vi "DecodeVireoToBotSpeak.vi"(3 "Via file":string="// Autogenerated Vireo assembly file\n// Generated on Wed Dec 18 16:11:37 2013\n\ndefine (c0, v(.UInt16 1) )\ndefine (c1, v(.UInt16 0) )\ndefine (c2, v(.UInt8 13) )\ndefine (c3, v(.Single 1000) )\n//---------------------------------------------------\n//VI Definition: Demo1.vi\ndefine (videf1, v(.VirtualInstrument, (\n    c(\n        e(.Utf8String local1)   // Reply\n        e(c(\n            e(.UInt8 n0)   // Numeric\n        ) local2)   // Info Out\n        e(.Utf8String local3)   // Reply\n        e(c(\n            e(.UInt8 n0)   // Numeric\n        ) local4)   // Info Out\n        e(.Utf8String local5)   // Reply\n    )\n    1,\n    clump(1,\n        videf2(c1 local1  c2 local2)\n        videf3( local3 local2  local4)\n        videf2(c0 local5 local4 c2 local2)\n//--- end of vi\n    )\n)))\n//---------------------------------------------------\n//VI Definition: DigitalWrite.vi\ndefine (videf2, v(.VirtualInstrument, (\n    c(\n        i(v(.UInt16 0) local4)   // State\n        o(v(.Utf8String '') local3)   // Reply\n        i(v(c(\n            e(.UInt8 n0)   // Numeric\n        ) (0 )) local1)   // Info In\n        i(v(.UInt8 0) local5)   // Port\n        o(v(c(\n            e(.UInt8 n0)   // Numeric\n        ) (0 )) local2)   // Info Out\n    )\n    c(\n        e(v(.Int32 -1) local6)\n    )\n    1,\n    clump(1,\n        Copy(local1 local2 )                      // FP Term\n//--- end of vi\n    )\n)))\n//---------------------------------------------------\n//VI Definition: VS_Wait.vi\ndefine (videf3, v(.VirtualInstrument, (\n    c(\n        i(v(.Single 1) local4)   // delay (s)\n        o(v(.Utf8String '') local3)   // Reply\n        i(v(c(\n            e(.UInt8 n0)   // Numeric\n        ) (0 )) local1)   // Info In\n        i(v(.UInt8 0) local8)   // Timer\n        o(v(c(\n            e(.UInt8 n0)   // Numeric\n        ) (0 )) local2)   // Info Out\n    )\n    c(\n        e(.Single local5)\n        e(.UInt32 local6)   // milliseconds to wait\n        e(.UInt32 local7)   // millisecond timer value\n        e(v(.Int32 -1) local9)\n    )\n    1,\n    clump(1,\n        Copy(local1 local2 )                      // FP Term\n        Mul(local4 c3 local5)\n        Convert(local5 local6)\n        WaitMilliseconds(local6)\n//--- end of vi\n    )\n)))\nenqueue (videf1)\n") -> (1 "BotSpeak":string)   [LabVIEW 2012]
panel:
  out "Array 3":string[](array[string])
  out "Params":cluster{"Constant":string, "value":string}[](array[cluster])
  out "Array":T1(array[cluster])
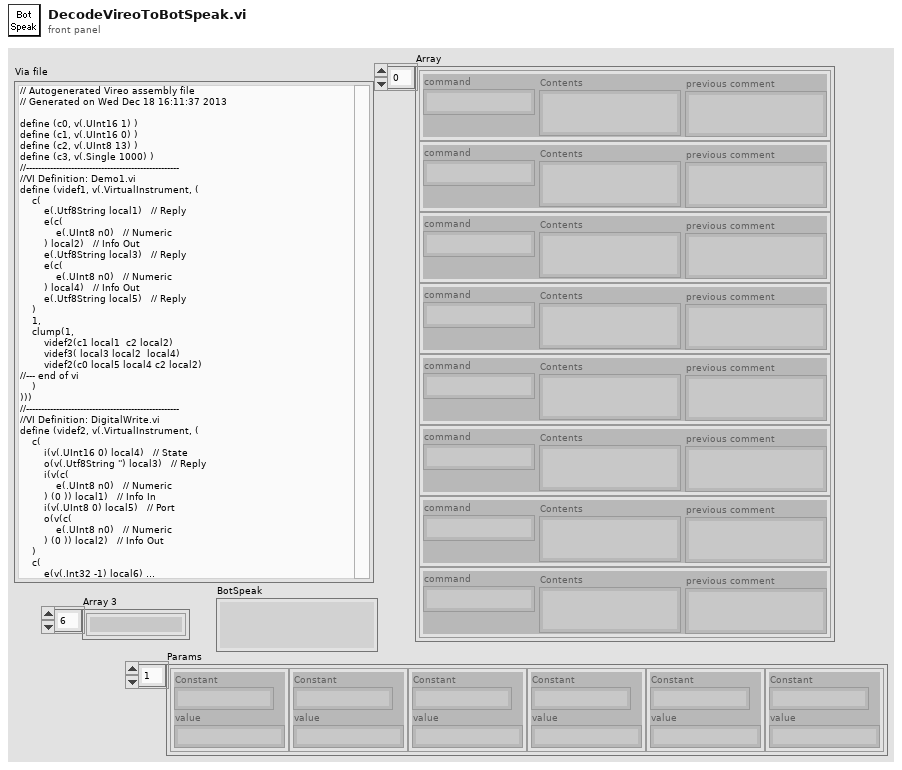
[diagram p1: front panel]
types:
  T1 = cluster{"command":string, "Contents":string, "previous comment":string}[]
  T2 = cluster{"Contents":string, "Contents 2":string}[]
  T3 = cluster{"command":string, "Contents":string, "Via file":string}
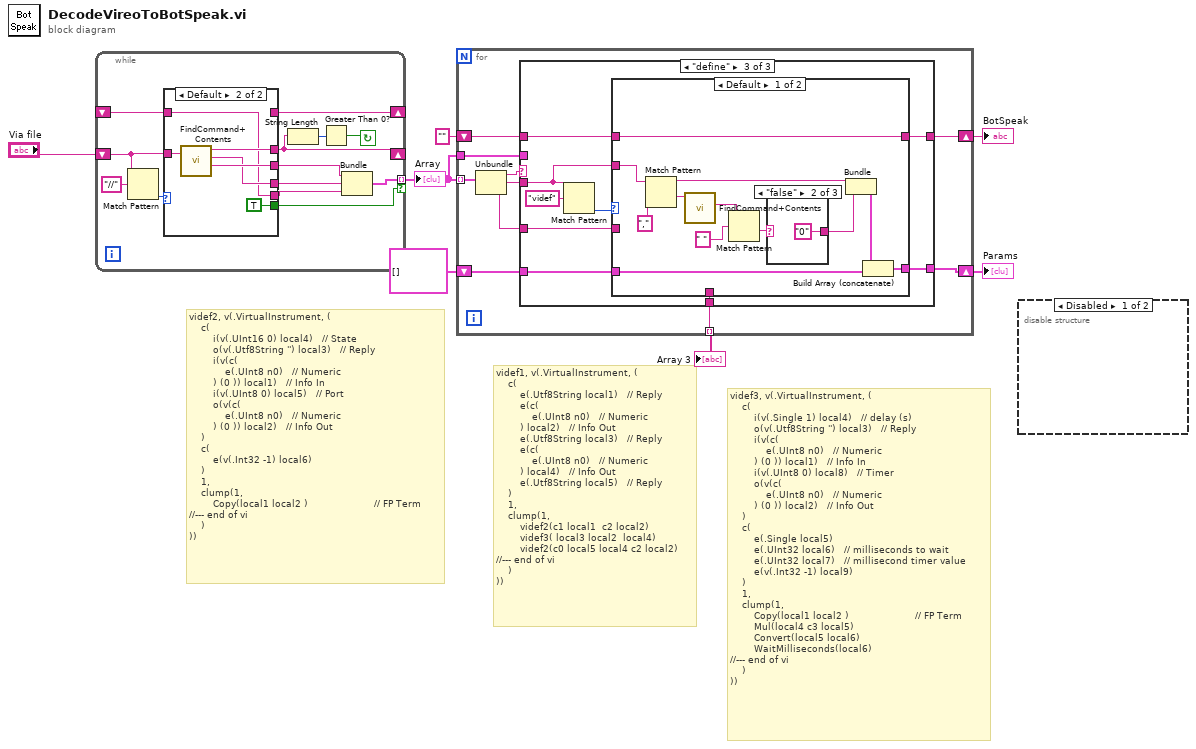
[diagram p0: block diagram]
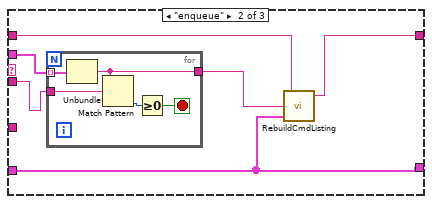
[diagram p4: hidden frame]
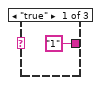
[diagram p5: hidden frame]
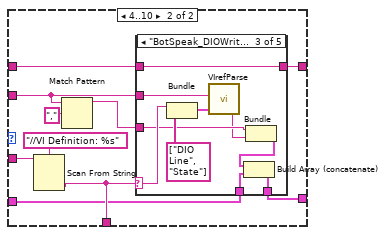
[diagram p7: hidden frame]
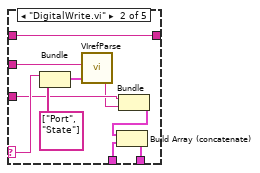
[diagram p9: hidden frame]
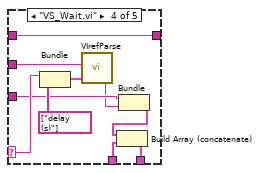
[diagram p10: hidden frame]
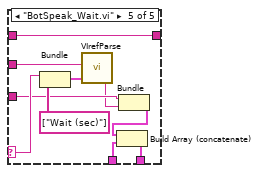
[diagram p11: hidden frame]
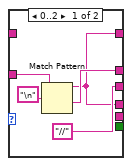
[diagram p12: hidden frame]
diagram:
  # "videf3, v(.VirtualInstrument, (\n    c(\n        i(v(.Single 1) local4)   // delay (s)\n        o(v(.Utf8String '') local3)   // Reply\n        i(v(c(\n            e(.UInt8 n0)   // Numeric\n        ) (0 )) local1)   // Info In\n        i(v(.UInt8 0) local8)   // Timer\n        o(v(c(\n            e(.UInt8 n0)   // Numeric\n        ) (0 )) local2)   // Info Out\n    )\n    c(\n        e(.Single local5)\n        e(.UInt32 local6)   // milliseconds to wait\n        e(.UInt32 local7)   // millisecond timer value\n        e(v(.Int32 -1) local9)\n    )\n    1,\n    clump(1,\n        Copy(local1 local2 )                      // FP Term\n        Mul(local4 c3 local5)\n        Convert(local5 local6)\n        WaitMilliseconds(local6)\n//--- end of vi\n    )\n))"
  # "videf1, v(.VirtualInstrument, (\n    c(\n        e(.Utf8String local1)   // Reply\n        e(c(\n            e(.UInt8 n0)   // Numeric\n        ) local2)   // Info Out\n        e(.Utf8String local3)   // Reply\n        e(c(\n            e(.UInt8 n0)   // Numeric\n        ) local4)   // Info Out\n        e(.Utf8String local5)   // Reply\n    )\n    1,\n    clump(1,\n        videf2(c1 local1  c2 local2)\n        videf3( local3 local2  local4)\n        videf2(c0 local5 local4 c2 local2)\n//--- end of vi\n    )\n))"
  # "videf2, v(.VirtualInstrument, (\n    c(\n        i(v(.UInt16 0) local4)   // State\n        o(v(.Utf8String '') local3)   // Reply\n        i(v(c(\n            e(.UInt8 n0)   // Numeric\n        ) (0 )) local1)   // Info In\n        i(v(.UInt8 0) local5)   // Port\n        o(v(c(\n            e(.UInt8 n0)   // Numeric\n        ) (0 )) local2)   // Info Out\n    )\n    c(\n        e(v(.Int32 -1) local6)\n    )\n    1,\n    clump(1,\n        Copy(local1 local2 )                      // FP Term\n//--- end of vi\n    )\n))"
  n1 = while {
    shift-right: [w20] -> _
    shift-left: "Via file" -> [w14]
    tunnel: [w15] -> w1 mode=indexing if=w9
    shift-right: [w11] -> _
    shift-left: _ -> [w10]
    stop <- w18 continue-if-true
    n2 = Match Pattern(string=w14, regular expression="//") -> (offset past match=w12:i32)  [unwired: 1 in, 3 out]
    n3 = case shown="Default" w12 {
      tunnel: [w23 w31] -> w20
      tunnel: ["//" ("regular expression") w30] -> w17
      tunnel: [w21 w29] -> w16
      tunnel: w14 -> [w25 w28]
      tunnel: [w21 _] -> w11
      tunnel: [_ w27] -> w8
      tunnel: w10 -> [_ w27]
      tunnel: [_ TRUE] -> w9
      frame 0..2 {
        n4 = Match Pattern(string=w25, regular expression="\n") -> (before substring=w21:string, after substring=w23:string)  [unwired: 1 in, 2 out]
      }
      frame Default {
        n5 = call "FindCommand+Contents.vi"("Via file in"=w28) -> ("left"=w31:string, "Contents"=w29:string, "command"=w30:string)  [unwired: 1 in, 1 out]
      }
    }
    n6 = String Length(string=w20) -> (length=w19:i32)
    n7 = Greater Than 0?(x=w19) -> (x > 0?=w18:bool)
    n8 = Bundle("command"=w17, "Contents"=w16, "Via file"=w8) -> (w15:T3)  [unwired: 1 in]
  }
  "Array" <- w1
  n9 = for {
    tunnel: w1 -> [w41] mode=indexing
    shift-right: [w36] -> w5
    shift-left: "" -> [w37]
    shift-right: [w35] -> w3
    shift-left: T2 [] -> [w34]
    tunnel: [w33] -> w2 mode=indexing
    tunnel: w1 -> [w32]
    n10 = Unbundle(w41) -> ("command"=w40:string, "Contents"=w39:string, "Via file"=w38:string)
    n11 = case shown="\"define\"" w40 {
      tunnel: w39 -> [_ w46 w58]
      tunnel: w38 -> [_ _ w61]
      tunnel: w37 -> [w43 w48 w60]
      tunnel: [w43 w49 w59] -> w36
      tunnel: [w42 w44 w57] -> w35
      tunnel: w34 -> [w42 w44 w56]
      tunnel: [_ _ w55] -> w33
      tunnel: w32 -> [_ w47 _]
      frame Default {
      }
      frame "enqueue" {
        n12 = for {
          tunnel: w47 -> [w54] mode=indexing
          tunnel: w46 -> [w53]
          tunnel: [w50] -> w45
          stop <- w51 stop-if-true
          n13 = Unbundle(w54) -> ("Contents"=w50:string)  [unwired: 2 out]
          n14 = Match Pattern(string=w50, regular expression=w53) -> (offset past match=w52:i32)  [unwired: 1 in, 3 out]
          n15 = Greater Or Equal To 0?(x=w52) -> (x >= 0?=w51:bool)
        }
        n16 = call "RebuildCmdListing.vi"("Params"=w44, "Contents"=w45, "String in"=w48) -> ("String out"=w49:string)  [unwired: 1 in, 1 out]
      }
      frame "define" {
        n17 = Match Pattern(string=w58, regular expression="videf") -> (offset past match=w62:i32)  [unwired: 1 in, 3 out]
        n18 = case shown="Default" w62 {
          tunnel: w61 -> [_ w88]
          tunnel: w60 -> [w75 w86]
          tunnel: [w75 w85] -> w59
          tunnel: w58 -> [w73 w83]
          tunnel: [w67 w79] -> w57
          tunnel: w56 -> [w66 w80]
          tunnel: [_ w84] -> w55
          frame Default {
            n19 = Match Pattern(string=w73, regular expression=",") -> (before substring=w71:string, after substring=w72:string)  [unwired: 1 in, 2 out]
            n20 = call "FindCommand+Contents.vi"("Via file in"=w72) -> ("Contents"=w70:string)  [unwired: 1 in, 3 out]
            n21 = Match Pattern(string=w70, regular expression=" ") -> (after substring=w65:string)  [unwired: 1 in, 3 out]
            n22 = case shown="\"false\"" w65 {
              selector: w65 -> [_ _ w78]
              tunnel: ["1" "0" w78] -> w64
              frame "true" {
              }
              frame "false" {
              }
              frame Default {
              }
            }
            n23 = Bundle("Contents"=w71, w64) -> (w68:cluster{"Contents":string, string})  [unwired: 1 in]
            n24 = Build Array (concatenate)(w68, w66) -> (w67:T2)
          }
          frame 4..10 {
            n25 = Scan From String(format string="//VI Definition: %s" ("regular expression"), input string=w88) -> (output 1=w84:string)  [unwired: 3 in, 3 out]
            n26 = Match Pattern(string=w83, regular expression=",") -> (before substring=w81:string)  [unwired: 1 in, 3 out]
            n27 = case shown="\"BotSpeak_DIOWrite.vi\"" w84 {
              selector: w84 -> [_ w99 w109 w119 w129]
              tunnel: w86 -> [w90 w96 w106 w116 w126]
              tunnel: [w90 w96 w106 w116 w126] -> w85
              tunnel: w83 -> [_ w100 w110 w120 w130]
              tunnel: w81 -> [_ w95 w105 w115 w125]
              tunnel: w80 -> [w89 w92 w102 w112 w122]
              tunnel: [w89 w91 w101 w111 w121] -> w79
              frame Default {
              }
              frame "DigitalWrite.vi" {
                n28 = Bundle(w99, string[] ["Port", "State"]) -> (w97:cluster{string, string[]})  [unwired: 1 in]
                n29 = call "VIrefParse.vi"("Params"=w97, "VIA"=w100) -> ("String out"=w94:string)  [unwired: 3 in]
                n30 = Bundle("Contents"=w95, "String out"=w94) -> (w93:cluster{"Contents":string, "String out":string})  [unwired: 1 in]
                n31 = Build Array (concatenate)(w93, w92) -> (w91:T2)
              }
              frame "BotSpeak_DIOWrite.vi" {
                n32 = Bundle(w109, string[] ["DIO Line", "State"]) -> (w107:cluster{string, string[]})  [unwired: 1 in]
                n33 = call "VIrefParse.vi"("Params"=w107, "VIA"=w110) -> ("String out"=w104:string)  [unwired: 3 in]
                n34 = Bundle("Contents"=w105, "String out"=w104) -> (w103:cluster{"Contents":string, "String out":string})  [unwired: 1 in]
                n35 = Build Array (concatenate)(w103, w102) -> (w101:T2)
              }
              frame "VS_Wait.vi" {
                n36 = Bundle(w119, string[] ["delay (s)"]) -> (w117:cluster{string, string[]})  [unwired: 1 in]
                n37 = call "VIrefParse.vi"("Params"=w117, "VIA"=w120) -> ("String out"=w114:string)  [unwired: 3 in]
                n38 = Bundle("Contents"=w115, "String out"=w114) -> (w113:cluster{"Contents":string, "String out":string})  [unwired: 1 in]
                n39 = Build Array (concatenate)(w113, w112) -> (w111:T2)
              }
              frame "BotSpeak_Wait.vi" {
                n40 = Bundle(w129, string[] ["Wait (sec)"]) -> (w127:cluster{string, string[]})  [unwired: 1 in]
                n41 = call "VIrefParse.vi"("Params"=w127, "VIA"=w130) -> ("String out"=w124:string)  [unwired: 3 in]
                n42 = Bundle("Contents"=w125, "String out"=w124) -> (w123:cluster{"Contents":string, "String out":string})  [unwired: 1 in]
                n43 = Build Array (concatenate)(w123, w122) -> (w121:T2)
              }
            }
          }
        }
      }
    }
  }
  "BotSpeak" <- w5
  "Params" <- w3
  "Array 3" <- w2
  n44 = disable-structure shown="Disabled" {
    frame Disabled {
    }
    frame Enabled {
    }
  }
